vi "Bundle Test Data.vi"(4 "force time":dbl[](array[numeric]), 5 "array results in":T1, 6 "setpoint":dbl[](array[numeric]), 7 "servo pw":dbl[](array[numeric]), 9 "force":dbl[](array[numeric]), 10 "diameter":dbl[](array[numeric]), 11 "diameter time":dbl[](array[numeric])) -> (3 "array results out":T1)   [LabVIEW 2020]
uses:
  Controller Loop/Controller Data.ctl
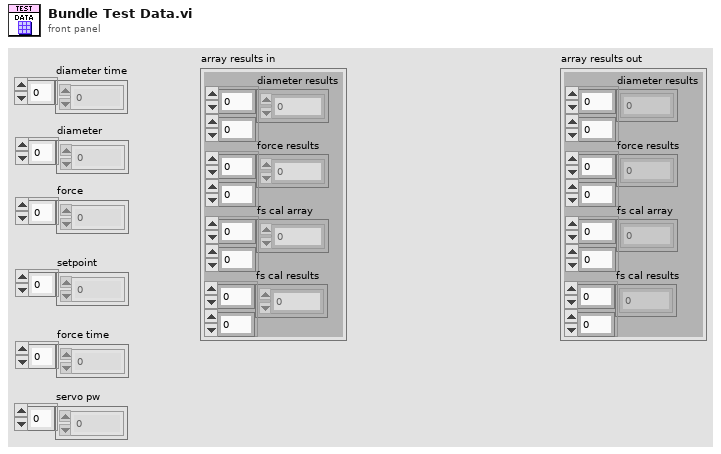
[diagram p1: front panel]
types:
  T1 = typedef "Controller Data.ctl" = cluster{"diameter results":dbl[][], "force results":dbl[][], "fs cal array":dbl[][], "fs cal results":dbl[][]}
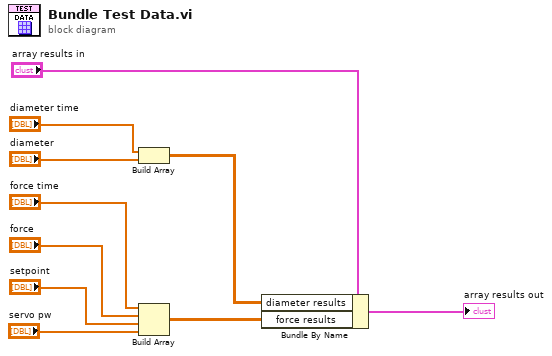
[diagram p0: block diagram]
diagram:
  n1 = Build Array("diameter time", "diameter") -> (w4:dbl[][])
  n2 = Build Array("force time", "force", "setpoint", "servo pw") -> (w3:dbl[][])
  n3 = Bundle By Name(cluster="array results in", "diameter results"=w4, "force results"=w3) -> (→"array results out":T1)
